vi "check for sequential tags.vi"(11 "indices in":i32[](array[numeric])) -> (1 "first index":i32, 2 "sequential?":bool, 3 "indices out":i32[](array[numeric]))   [LabVIEW 2014, in "Shared Memory runtime.lvclass"]
uses:
  Shared Memory runtime.lvclass
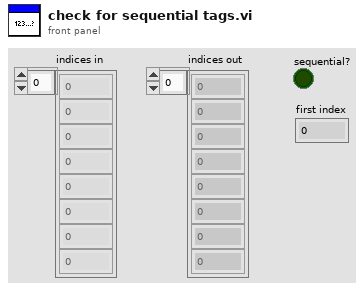
[diagram p1: front panel]
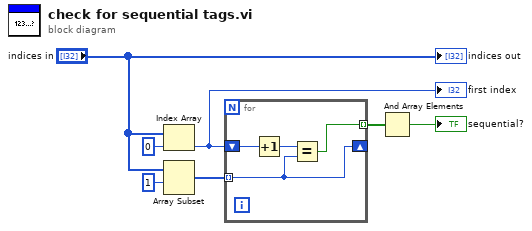
[diagram p0: block diagram]
diagram:
  n1 = Index Array(array="indices in", index=0) -> (element=w4:i32)
  "first index" <- w4
  n2 = Array Subset(array="indices in", index=1) -> (w3:i32[])  [unwired: 1 in]
  n3 = for {
    shift-right: [w11] -> _
    shift-left: w4 -> [w10]
    tunnel: w3 -> [w11] mode=indexing
    tunnel: [w8] -> w2 mode=indexing
    n4 = Increment(x=w10) -> (x+1=w9:i32)
    n5 = Equal?(x=w9, y=w11) -> (x = y?=w8:bool)
  }
  n6 = And Array Elements(Boolean array=w2) -> (logical AND=→"sequential?":bool)
  "indices out" <- "indices in"
